vi "Write B.vi"(8 "error in (no error)":errorcluster, 10 "B":dbl, 11 "Divide in":refnum<class "Divide.lvclass">) -> (0 "error out":errorcluster, 3 "Divide out":refnum<class "Divide.lvclass">)   [LabVIEW 2023, in "Divide.lvclass"]
uses:
  Divide.lvclass
  Divide.lvclass/Divide.ctl
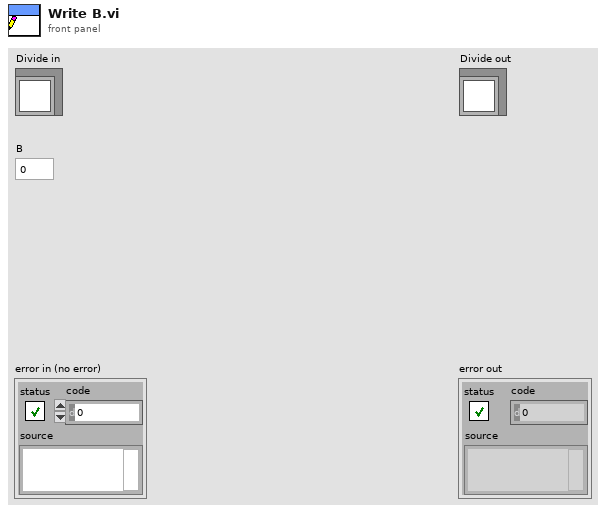
[diagram p1: front panel]
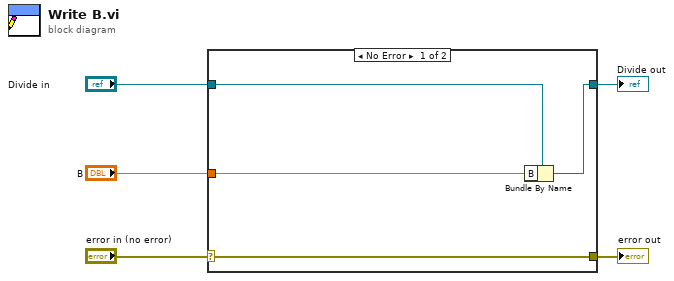
[diagram p0: block diagram]
diagram:
  n1 = case shown="No Error" "error in (no error)" {
    selector: "error in (no error)" -> [w9 w10]
    tunnel: [w9 w10] -> w4
    tunnel: [w7 w11] -> w2
    tunnel: "Divide in" -> [w8 w11]
    tunnel: "B" -> [w6 _]
    frame No Error {
      n2 = Bundle By Name(cluster=w8, "B"=w6) -> (w7:refnum<class "Divide.lvclass">)
    }
    frame Error {
    }
  }
  "error out" <- w4
  "Divide out" <- w2
